vi "Rohde & Schwarz VNA Convert Form 2 Data.vi"(8 "Raw Data Point":string) -> (0 "Number":cdb)   [LabVIEW 2011]
panel:
  out "Single Array":sgl[](array[numeric])
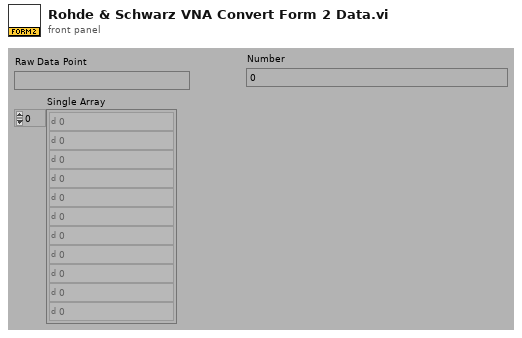
[diagram p1: front panel]
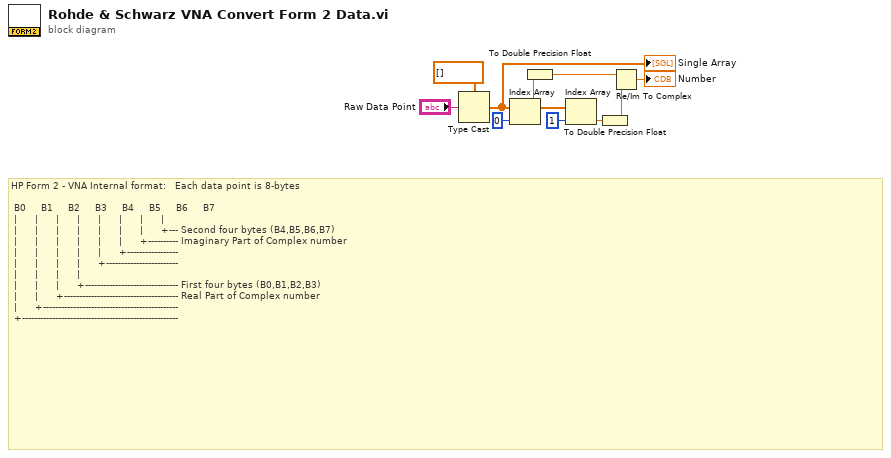
[diagram p0: block diagram]
diagram:
  # "HP Form 2 - VNA Internal format:   Each data point is 8-bytes\n\n B0     B1     B2     B3     B4     B5     B6     B7\n |      |      |      |      |      |      |      |\n |      |      |      |      |      |      |      +--- Second four bytes (B4,B5,B6,B7)\n |      |      |      |      |      |      +---------- Imaginary Part of Complex number\n |      |      |      |      |      +-----------------\n |      |      |      |      +------------------------\n |      |      |      |\n |      |      |      +------------------------------- First four bytes (B0,B1,B2,B3)\n |      |      +-------------------------------------- Real Part of Complex number\n |      +---------------------------------------------\n +----------------------------------------------------"
  n1 = Type Cast(type=sgl[] [], x="Raw Data Point") -> (*(type *) &x=w1:sgl[])
  "Single Array" <- w1
  n2 = Index Array(array=w1, index=0) -> (element=w4:sgl)
  n3 = To Double Precision Float(number=w4) -> (double precision float=w3:dbl)
  n4 = Index Array(array=w1, index=1) -> (element=w6:sgl)
  n5 = To Double Precision Float(number=w6) -> (double precision float=w5:dbl)
  n6 = Re/Im To Complex(1:w5, 2:w3) -> (0:→"Number":cdb)
